vi "Get settings chain.vi"(8 "error in (no error)":errorcluster, 11 "TemplateBase in":refnum<class "BMC.lvclass">) -> (0 "error out":errorcluster, 1 "class name":string[](array[string]), 2 "settings":variant[](array[variant]), 3 "TemplateBase out":refnum<class "BMC.lvclass">)   [LabVIEW 2012, in "BMC.lvclass"]
doc: "Returns an array of variants containing the settings clusters of each class in the inheritance chain (lowest child class first), together with an array of all class names in the inheritance chain.\n\nFor classes without settings cluster, the settings chain contains empty variants."
uses:
  BMC.lvclass
  <vilib>/Distrio/Murmex/Murmex/Murmex.lvclass
  BMC.lvclass/BMC.ctl
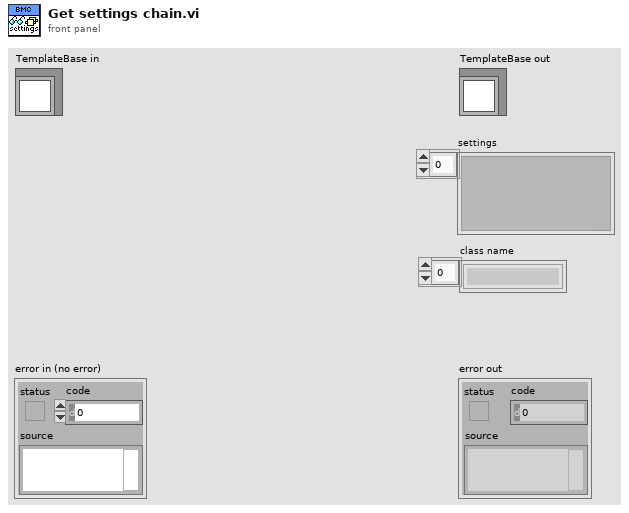
[diagram p1: front panel]
types:
  T1 = typedef "BMC.lvclass/settings_cluster.ctl" = cluster{"Voltage Map file":path, "Superactuator":dbl, "Optimisation name":string, "Starting shape":T2}
  T2 = typedef "BMC.lvclass/starting shape.ctl" = enum16{"Start from Mid range", "Load starting shape"}
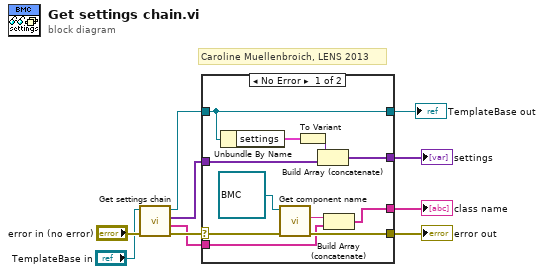
[diagram p0: block diagram]
diagram:
  # "Caroline Muellenbroich, LENS 2013"
  n1 = call-parent "Get settings chain.vi"("error in (no error)"="error in (no error)", "MurmexBase in"="TemplateBase in") -> ("error out"=w8:errorcluster, "class name"=w6:string[], "settings"=w2:variant[], "MurmexBase out"=w4:refnum<class "BMC.lvclass">)  [unwired: 6 in]
  n2 = case shown="No Error" w8 {
    selector: w8 -> [w21 w23]
    tunnel: [w19 w23] -> w7
    tunnel: w6 -> [w17 w22]
    tunnel: [w16 w22] -> w5
    tunnel: w4 -> [w11 w25]
    tunnel: [w13 w24] -> w3
    tunnel: w2 -> [w12 w24]
    tunnel: [w11 w25] -> w1
    frame No Error {
      n3 = Unbundle By Name(w11) -> ("settings"=w14:T1)
      n4 = call <vilib>:"Get component name.vi"("error in (no error)"=w21, "Murmex in"=refnum<class "BMC.lvclass"> refnum ("BMC")) -> ("error out"=w19:errorcluster, "component name"=w18:string)  [unwired: 7 in, 1 out]
      n5 = To Variant(anything=w14) -> (Variant=w15:variant)
      n6 = Build Array (concatenate)(w15, w12) -> (w13:variant[])
      n7 = Build Array (concatenate)(w18, w17) -> (w16:string[])
    }
    frame Error {
    }
  }
  "error out" <- w7
  "TemplateBase out" <- w1
  "settings" <- w3
  "class name" <- w5
